vi "sv_Octave Band Frequencies.vi"(0 "octave band selector":i32, 1 "reference frequency range":u16(ring)=1 items=["Infrasonic", "Audio", "Ultrasonic"], 4 "bandwidth":T2(ring)=enum."1/3 octave", 5 "standard":T1) -> (2 "reference frequency [Hz]":dbl format="%.2f", 3 "bandedge frequencies [Hz]":cluster{"f low":dbl, "f high":dbl} {"f high" format="%.2f"; "f low" format="%.2f"}, 6 "bandwidth designator":dbl format="%.2f", 7 "midband frequency [Hz]":dbl format="%.2f")   [LabVIEW 2017, in "SoundVib_Octave.lvlib"]
doc: "Returns the midband and bandedge frequencies associated with a particular fractional-octave band based on the specified bandwidth and standard (ANSI or IEC).\nThe octave band selector specifies the fractional-octave band. A value of 0 corresponds to the reference frequency of the audio-frequency range, 1 kHz. Each successive value corresponds to the next fractional-octave band. Positive values cover the range above 1 kHz, and negative values cover the range below 1 kHz."
uses:
  <vilib>/addons/Sound and Vibration/svt_Octave/SoundVib_Octave.lvlib
  <vilib>/addons/_NISVFA/_Shared subVIs/Controls/svc_Octave Standard.ctl
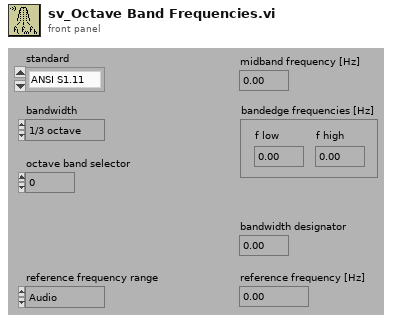
[diagram p1: front panel]
types:
  T1 = typedef "svc_Octave Standard.ctl" = enum16{"ANSI S1.11", "IEC 61260"}
  T2 = enum16{"1 octave", "1/3 octave", "1/6 octave", "1/12 octave", "1/24 octave", "1/48 octave", "1/96 octave"}
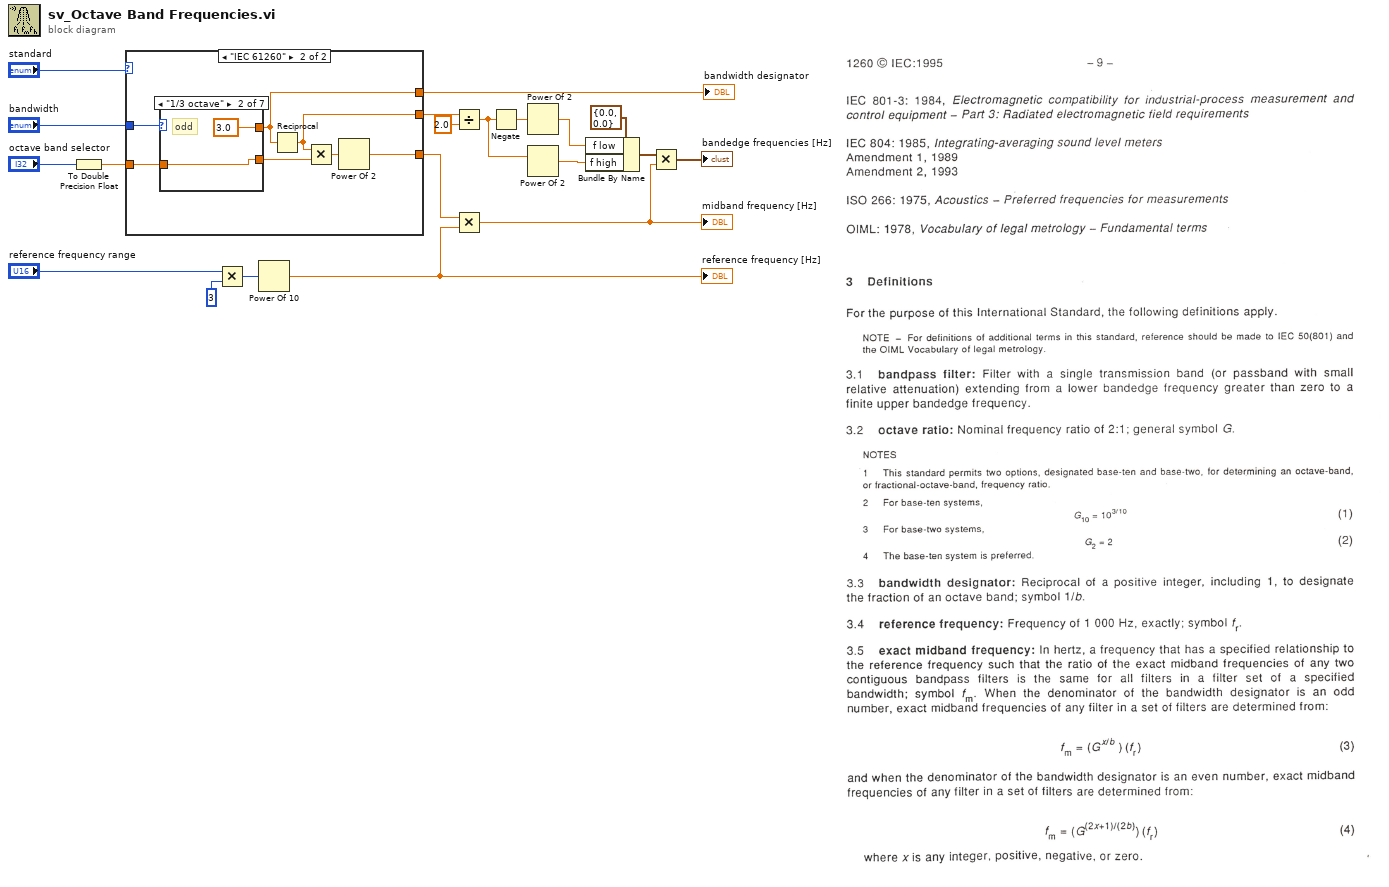
[diagram p0: block diagram]
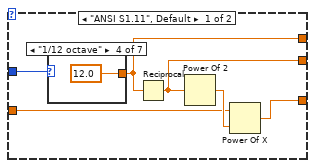
[diagram p2: hidden frame]
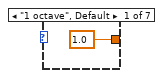
[diagram p3: hidden frame]
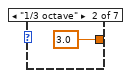
[diagram p4: hidden frame]
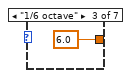
[diagram p5: hidden frame]
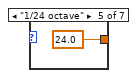
[diagram p6: hidden frame]
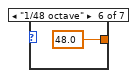
[diagram p7: hidden frame]
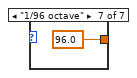
[diagram p8: hidden frame]
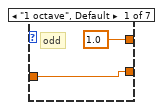
[diagram p9: hidden frame]
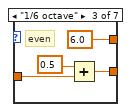
[diagram p10: hidden frame]
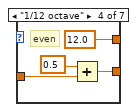
[diagram p11: hidden frame]
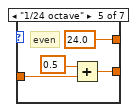
[diagram p12: hidden frame]
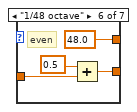
[diagram p13: hidden frame]
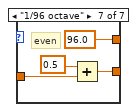
[diagram p14: hidden frame]
diagram:
  n1 = To Double Precision Float(number="octave band selector") -> (double precision float=w1:dbl)
  n2 = case shown="\"IEC 61260\"" "standard" {
    tunnel: "bandwidth" -> [w25 w40]
    tunnel: w1 -> [w24 w39]
    tunnel: [w23 w38] -> w4
    tunnel: [w21 w36] -> w18
    tunnel: [w22 w37] -> w6
    frame "ANSI S1.11", Default {
      n3 = case shown="\"1/12 octave\"" w25 {
        tunnel: [1.0 ("x") 3.0 ("x") 6.0 ("x") 12.0 ("x") 24.0 ("x") 48.0 ("x") 96.0 ("x")] -> w21
        frame "1 octave", Default {
        }
        frame "1/3 octave" {
        }
        frame "1/6 octave" {
        }
        frame "1/12 octave" {
        }
        frame "1/24 octave" {
        }
        frame "1/48 octave" {
        }
        frame "1/96 octave" {
        }
      }
      n4 = Reciprocal(x=w21) -> (1/x=w22:dbl)
      n5 = Power Of 2(x=w22) -> (2^x=w26:dbl)
      n6 = Power Of X(1:w26, 2:w24) -> (0:w23:dbl)
    }
    frame "IEC 61260" {
      n7 = case shown="\"1/3 octave\"" w40 {
        tunnel: [1.0 ("x") 3.0 ("x") 6.0 ("x") 12.0 ("x") 24.0 ("x") 48.0 ("x") 96.0 ("x")] -> w36
        tunnel: w39 -> [w41 w43 w47 w50 w54 w58 w62]
        tunnel: [w41 w43 w45 w49 w53 w57 w61] -> w35
        frame "1 octave", Default {
          # "odd"
        }
        frame "1/3 octave" {
          # "odd"
        }
        frame "1/6 octave" {
          # "even"
          n8 = Add(x=0.5, y=w47) -> (x+y=w45:dbl)
        }
        frame "1/12 octave" {
          # "even"
          n9 = Add(x=0.5, y=w50) -> (x+y=w49:dbl)
        }
        frame "1/24 octave" {
          # "even"
          n10 = Add(x=0.5, y=w54) -> (x+y=w53:dbl)
        }
        frame "1/48 octave" {
          # "even"
          n11 = Add(x=0.5, y=w58) -> (x+y=w57:dbl)
        }
        frame "1/96 octave" {
          # "even"
          n12 = Add(x=0.5, y=w62) -> (x+y=w61:dbl)
        }
      }
      n13 = Reciprocal(x=w36) -> (1/x=w37:dbl)
      n14 = Multiply(x=w37, y=w35) -> (x*y=w34:dbl)
      n15 = Power Of 2(x=w34) -> (2^x=w38:dbl)
    }
  }
  "bandwidth designator" <- w18
  n16 = Multiply(x="reference frequency range", y=u16 3) -> (x*y=w16:u16)
  n17 = Power Of 10(x=w16) -> (10^x=w3:dbl)
  "reference frequency [Hz]" <- w3
  n18 = Divide(x=w6, y=2.0) -> (x/y=w8:dbl)
  n19 = Multiply(x=w4, y=w3) -> (x*y=w2:dbl)
  "midband frequency [Hz]" <- w2
  n20 = Negate(x=w8) -> (-x=w9:dbl)
  n21 = Power Of 2(x=w9) -> (2^x=w12:dbl)
  n22 = Power Of 2(x=w8) -> (2^x=w11:dbl)
  n23 = Bundle By Name(cluster=cluster{"f low":dbl, "f high":dbl} {"f low"=0.0, "f high"=0.0} ("bandedge frequencies [Hz] 2"), "f low"=w12, "f high"=w11) -> (w10:cluster{"f low":dbl, "f high":dbl})
  n24 = Multiply(x=w10, y=w2) -> (x*y=→"bandedge frequencies [Hz]":cluster{"f low":dbl, "f high":dbl})
